vi "Multiple(SubVI).vi"(10 "y":dbl, 11 "x":dbl) -> (3 "Numeric":dbl)   [LabVIEW 2021]
doc: "Mutiple Two Numbers"
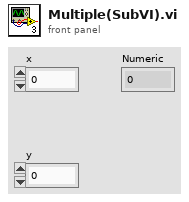
[diagram p1: front panel]
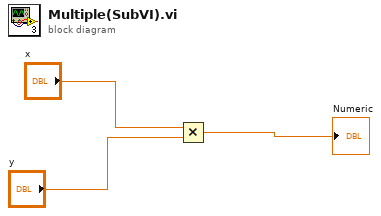
[diagram p0: block diagram]
diagram:
  n1 = Multiply(x="x", y="y") -> (x*y=→"Numeric":dbl)
